vi "Mode Array SLM.vi"(2 "Action":u16(ring) items=["Read", "Initialize"]) -> (8 "mode array":dbl[][][](array[numeric]))   [LabVIEW 2014]
uses:
  <vilib>/Utility/file.llb/Read From Spreadsheet File (DBL).vi
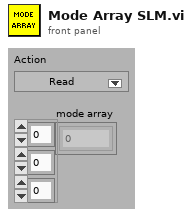
[diagram p1: front panel]
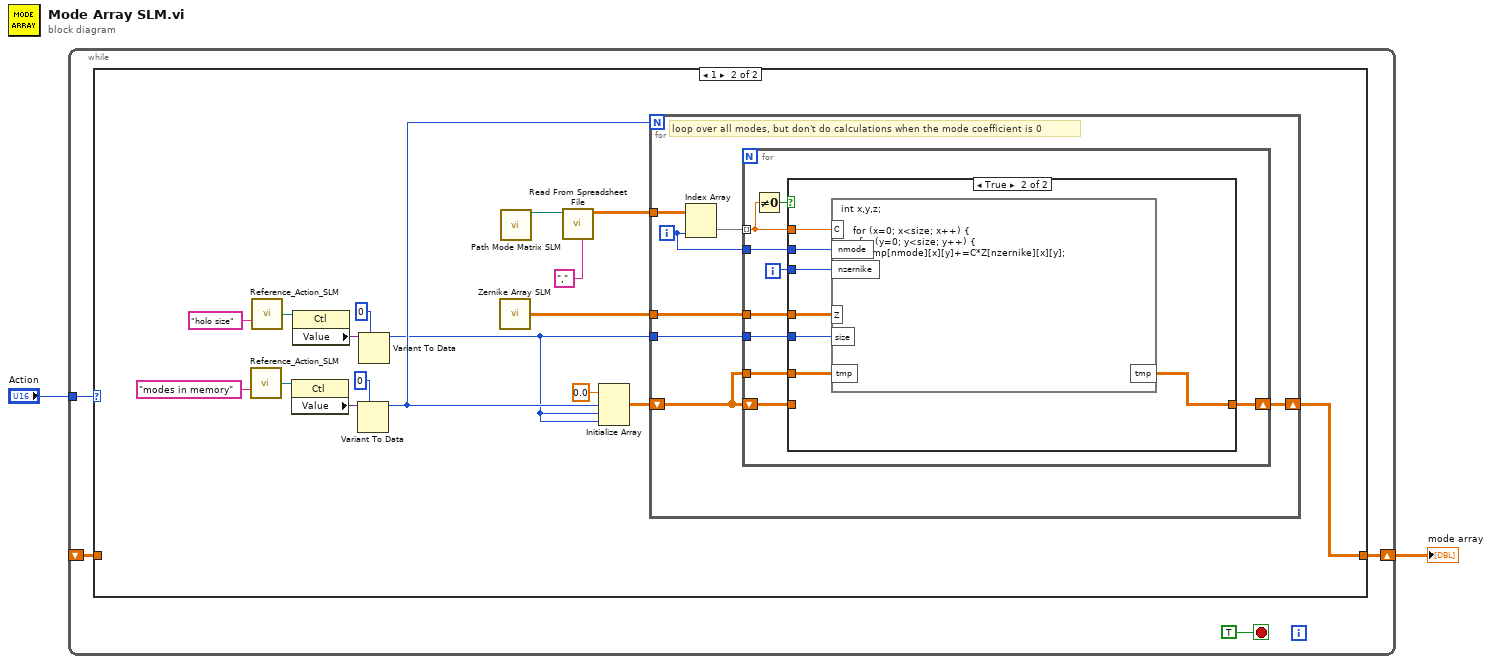
[diagram p0: block diagram]
diagram:
  n1 = while {
    shift-right: [w3] -> w1
    shift-left: _ -> [w4]
    tunnel: "Action" -> [w5]
    stop <- TRUE stop-if-true
    n2 = case shown="1" w5 {
      tunnel: w4 -> [w7 _]
      tunnel: [w7 w13] -> w3
      frame 0, Default {
      }
      frame 1 {
        n3 = call "Reference_Action_SLM.vi"("Control Name"="modes in memory") -> ("Ref OUT"=w19:refnum<vi>)  [unwired: 12 in, 2 out]
        n4 = call "Reference_Action_SLM.vi"("Control Name"="holo size") -> ("Ref OUT"=w11:refnum<vi>)  [unwired: 12 in, 2 out]
        n5 = property class="Ctl"(reference=w19) -> ("Value"=w20:variant)  [unwired: 1 in, 2 out]
        n6 = property class="Ctl"(reference=w11) -> ("Value"=w10:variant)  [unwired: 1 in, 2 out]
        n7 = Variant To Data(type=0, Variant=w20) -> (data=w24:i32)  [unwired: 1 in, 1 out]
        n8 = Variant To Data(type=0, Variant=w10) -> (data=w8:i32)  [unwired: 1 in, 1 out]
        n9 = call "Zernike Array SLM.vi"() -> ("zernike array"=w14:dbl[][][])  [unwired: 15 in]
        n10 = call "Path Mode Matrix SLM.vi"() -> ("mode matrix path"=w16:path)  [unwired: 15 in]
        n11 = call-poly <vilib>:"Read From Spreadsheet File.vi"("delimiter (\\t)"="," ("delimiter (\\t)"), "file path (dialog if empty)"=w16) -> ("all rows"=w23:dbl[][])  [unwired: 3 in, 6 out]
        n12 = Initialize Array(0.0 ("element"), w24, w8, w8) -> (w22:dbl[][][])
        n13 = for {
          N: w24 -> [_]
          tunnel: w23 -> [w30]
          tunnel: w8 -> [w29]
          tunnel: w14 -> [w28]
          shift-right: [w25] -> w13
          shift-left: w22 -> [w27]
          i -> [w26]
          # "loop over all modes, but don't do calculations when the mode coefficient is 0"
          n14 = Index Array(array=w30, index (col)=w26) -> (element=w31:dbl[])  [unwired: 1 in]
          n15 = for {
            shift-right: [w33] -> w25
            shift-left: w27 -> [w34]
            tunnel: w28 -> [w37]
            tunnel: w29 -> [w40]
            tunnel: w31 -> [w36] mode=indexing
            tunnel: w27 -> [w39]
            tunnel: w26 -> [w32]
            i -> [w38]
            n16 = Not Equal To 0?(x=w36) -> (x != 0?=w35:bool)
            n17 = case shown="True" w35 {
              tunnel: w40 -> [_ w48]
              tunnel: w39 -> [_ w47]
              tunnel: w36 -> [_ w46]
              tunnel: w38 -> [_ w45]
              tunnel: w37 -> [_ w44]
              tunnel: w34 -> [w41 _]
              tunnel: [w41 w42] -> w33
              tunnel: w32 -> [_ w43]
              frame False {
              }
              frame True {
                n18 = formula code="int x,y,z;\n\n    for (x=0; x<size; x++) {\n      for (y=0; y<size; y++) {\n         tmp[nmode][x][y]+=C*Z[nzernike][x][y];\n      }\n   }"("C"=w46, "size"=w48, "tmp"=w47, "nzernike"=w45, "Z"=w44, "nmode"=w43) -> ("tmp"=w42:dbl[][][])
              }
            }
          }
        }
      }
    }
  }
  "mode array" <- w1
